vi "add Setup.vi"(8 "error in (no error)":errorcluster caption="Fehler (Eingang, kein Fehler)", 10 "Setup":refnum<class "Setup.lvclass">, 11 "Test Eingang":refnum<class "Norm.lvclass"> caption="DNL_LabVIEW Object in") -> (0 "error out":errorcluster caption="Fehler (Ausgang)", 3 "Test Ausgang":refnum<class "Norm.lvclass"> caption="DNL_LabVIEW Object out")   [LabVIEW 2013, in "DatenKlassen.lvlib" / "Norm.lvclass"]
doc: "Fügt einen Versuchsaufbau einer bestimmten Norm hinzu."
uses:
  Norm.lvclass
  Setup/Setup.lvclass
  Norm.lvclass/Norm.ctl
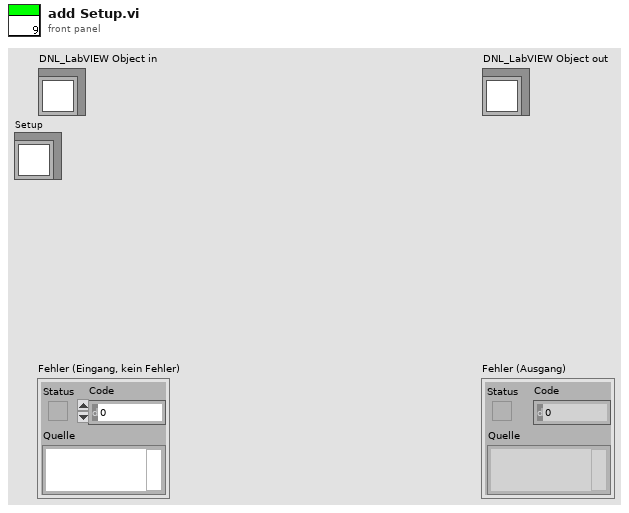
[diagram p1: front panel]
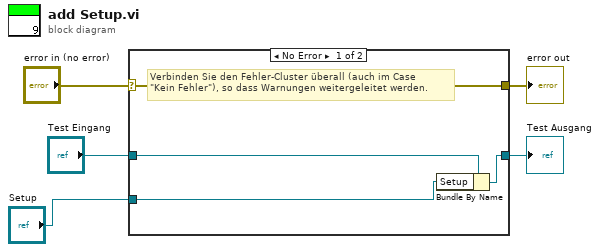
[diagram p0: block diagram]
diagram:
  n1 = case shown="No Error" "error in (no error)" {
    selector: "error in (no error)" -> [w9 w11]
    tunnel: [w9 w11] -> w4
    tunnel: [w7 w10] -> w2
    tunnel: "Test Eingang" -> [w8 w10]
    tunnel: "Setup" -> [w6 _]
    frame No Error {
      # "Verbinden Sie den Fehler-Cluster überall (auch im Case\n\"Kein Fehler\"), so dass Warnungen weitergeleitet werden."
      n2 = Bundle By Name(cluster=w8, "Setup"=w6) -> (w7:refnum<class "Norm.lvclass">)
    }
    frame Error {
    }
  }
  "error out" <- w4
  "Test Ausgang" <- w2
